vi "Get Number Devices.vi"(11 "numDevs":i32) -> (2 "function return":u32, 3 "numDevs out":i32)   [LabVIEW 2018, in "AndorSDK.lvlib"]
doc: "EXPNETTYPE unsigned int WINAPI GetNumberDevices(int * numDevs);"
uses:
  AndorSDK.lvlib
  ATMCD32D.dll
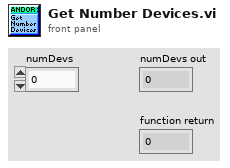
[diagram p1: front panel]
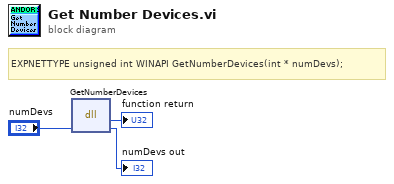
[diagram p0: block diagram]
diagram:
  # "EXPNETTYPE unsigned int WINAPI GetNumberDevices(int * numDevs);"
  n1 = dll-call lib="PTH2babs E\nPersönliches02 - Arbeit03-HiwijobsLabviewCodelibANDOR\tAndor SDK\nATMCD32D.*" fn="GetNumberDevices"("numDevs"="numDevs") -> (→"function return":u32, "numDevs"=→"numDevs out":i32)  [unwired: 3 in, 2 out]
